vi "calc_triangle_dist_average.vi"(1 "Array":dbl[][](array[numeric])) -> (0 "Numeric":dbl)   [LabVIEW 2011]
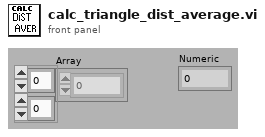
[diagram p1: front panel]
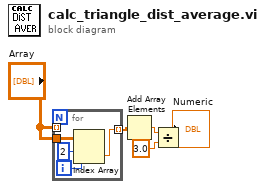
[diagram p0: block diagram]
diagram:
  n1 = for {
    tunnel: "Array" -> [w9]
    tunnel: [w7] -> w1 mode=indexing
    tunnel: "Array" -> [_] mode=indexing
    i -> [w6]
    n2 = Index Array(array=w9, index (row)=2 ("index"), index (col)=w6) -> (element=w7:dbl)
  }
  n3 = Add Array Elements(numeric array=w1) -> (sum=w3:dbl)
  n4 = Divide(x=w3, y=3.0) -> (x/y=→"Numeric":dbl)
